vi "GetAlazar_SaveToFile_25.vi"(0 "AlazarCluster":T12, 1 "Digitizer Settings":T8={"Digitizer delay (us) "=0.0, "rf points per line"=2048, "lines per plane"=128, "Samp Rate (Hz)"=100000000.0, "Additional dig delay (us)"=0.0, "Voltage Scale"=0.4, "Pre-Looks"=0, "Offset delay (us)"=0.0, "bits A/D"=8, "Avg Num"=1, "DigTimeOut"=5.0, "Rel Dig Delay"=0.0, "Dig Ch"=0, "LeCroyCluster"={"LeCroy Channels"=[TRUE, FALSE, FALSE, FALSE], "LC read pt offset"=0.0, "Sweep Avg"=FALSE}, "Main Digitizer"=enum."NI Digitizer", "Dig Config"=enum."Single channel", "Digitizer ID Cluster"={"Acqiris/Alazar/SP ID"=[], "NI Instr Handles"=[], "LeCroy VISA"="", "GaGe Handle"={"Handle"=0, "Sample size"=0, "Resolution"=0, "Offset"=0, "Channels"=0, "Boards"=0}, "ATS Ref"="ATS9350", "Acqiris Address"=["PCI::INSTR0"], "ADQRef"=refnum, "adq_cu_ptr"=refnum}, "Trigger Settings"={"Trig Source"=1, "Trig Coupling"=0, "Trig Slope"=0, "Level (mV)"=1500.0}, "Bulk Acq"=FALSE, "Bulk Start Indexes"=[], "Data Ref RF"=refnum, "NI ID/Channel"=[], "Total Dig CH"=1, "Xtra Ann Trig delay (us)"=10.0, "Fix Z Delay?"=FALSE, "One Way Transmission?"=FALSE, "Data Ref Log"=refnum} {"Trigger Settings"."Trig Slope" items=["Positive", "Negative"]; "Trigger Settings"."Level (mV)" format="%.2f"; "Trigger Settings"."Trig Coupling" items=["DC 1 MOhm", "AC 1 MOhm", "DC 50 Ohm", "AC 50 Ohm"]; "Trigger Settings"."Trig Source" items=["Chan 1", "External"]; "Rel Dig Delay" format="%.2f"; "DigTimeOut" format="%.2f"; "Avg Num" min=1; "Offset delay (us)" format="%.2f"; "Additional dig delay (us)" format="%.2f"; "Digitizer delay (us)" format="%.2f"}, 5 "Ann Array Params":T1={"Synth Foc?"=FALSE, "Focal Zones"=41, "Switch T/R"=0, "Trans Geometry (mm)"={"Transducer"=0, "Geo Focus"=12.0, "a (radius)"=3.0, "# of rings"=5, "kerf space "=0.1, "Center Freq"=12.0}, "Sub Ap Excite?"=FALSE, "Full Array Scan?"=FALSE, "Xmt/Rcv"={"XMIT"=[TRUE, TRUE, TRUE, TRUE, TRUE], "RCV"=[TRUE, TRUE, TRUE, TRUE, TRUE]}, "PulseSpacing (us)"=0.0, "Xmit Ring"=0, "XMIT CHS"=0, "RCV CHS"=0, "GPU?"=FALSE, "Save TIFF?"=FALSE, "downfactor"=1, "RCV 1CH"=0} {"RCV 1CH" items=["All", "1", "2", "3", "4", "5"]; "Trans Geometry (mm)"."Transducer" items=["6D 12R 40 MHz"=0, "10D 31R 20 MHz"=1, "10D 23R 20 MHz"=2, "6D 23R 40 MHz"=3, "4.5D 10.7R 40 MHz"=4, "9D 23.5R 20 MHz"=5, "9D 25.8R 20MHz"=6, "Enter"=99]; "Switch T/R" min=1 max=5 step=1}, 6 "Motion Settings":T4={"No Motion?"=FALSE, "Motion System"=enum."NI 735x", "Motion Bd ID"=1, "Motion Profile"="SMAC1", "# Axis"=1, "Reverse Z axis?"=TRUE, "SMAC Axis"=0, "scan pair"=enum."y-(x) scan", "RT fps"=6.0, "Steps per mm"=[1000, 1000, 1000, 1000], "Motor Parameters"={"velocity ct/s"=[10000.0, 10000.0, 10000.0, 50000.0], "accel ct/s^2"=[50000.0, 50000.0, 50000.0, 200000.0]}, "One Way Scan"=FALSE, "Reverse One Way Scan"=FALSE, "Global Position (mm)"=[], "Plane"=0, "Distance between\nscan lines (um)"=0.0, "Distance between\nscan planes (um)"=0.0, "number of scan planes"=1, "Total steps in line"=0, "Xtra plane\ndistance  (um)"=100, "Xtra planes "=1, "Add Axis"=FALSE, "overshoot cts"=200, "BKPT Shift"=0, "Scan Start Time (ms)"=0, "ESP VISA"="GPIB::1::INSTR", "3rd Axis"=1, "GL Ref Out"=refnum, "Galil Address"=""} {"3rd Axis" items=["x", "y", "z", "w"]; "Xtra planes" min=1; "Xtra plane\ndistance  (um)" min=0; "Distance between\nscan planes (um)" format="%.2f"; "Distance between\nscan lines (um)" format="%.2f"; "SMAC Axis" items=["None"=0, "Axis 1"=1, "Axis 2"=2, "Axis 3"=3, "Axis 4"=4, "Axis 5"=5, "Axis 6"=6, "Axis 7"=7, "Axis 8"=8, "Vector Space 1"=17, "Vector Space 2"=18, "Vector Space 3"=19, "Vector Space 4"=20]; "Motion Bd ID" min=1 max=32 step=1}, 7 "errorin":errorcluster, 8 "File Array":string[](array[string]), 10 "lines per plane":i32, 15 "Reverse?":bool) -> (17 "Raw VGain (scale)":dbl, 18 "Gain Array":T13(array[cluster]), 21 "VGain (dB)":dbl, 27 "error out":errorcluster)   [LabVIEW 2022 SP3]
uses:
  Motion Controllers/-MotionRoutines/MotionGlobals.vi
  -ScanSystem/DataHandling/ReverseData.vi
  -DigitizerRoutines/DigitizerSettings.ctl
  -DigitizerRoutines/DigitizerID.ctl
  -DigitizerRoutines/Digitizer.ctl
  Motion Controllers/NI_controller/-NI_MotionRoutines/MotionSys.ctl
  Motion Controllers/-MotionRoutines/ScanAxis.ctl
  Motion Controllers/NI_controller/-NI_MotionRoutines/MotionParameters.ctl
  Annular Array/-AnnularRoutines/ArrayGeometry.ctl
  Annular Array/-AnnularRoutines/TransGeometry.ctl
  Annular Array/-AnnularRoutines/AnnularArray.ctl
  -DigitizerRoutines/DigConfig.ctl
  Motion Controllers/-MotionRoutines/3rdAxis.ctl
  C:/Windows/System32/ADQAPI_dotNet_helper.dll
panel:
  in  "Channel (0) 2":i32
  out "read time":u32
  out "save time":u32
  out "Numeric":i32
  # "1-D and 2-D B scan settings"
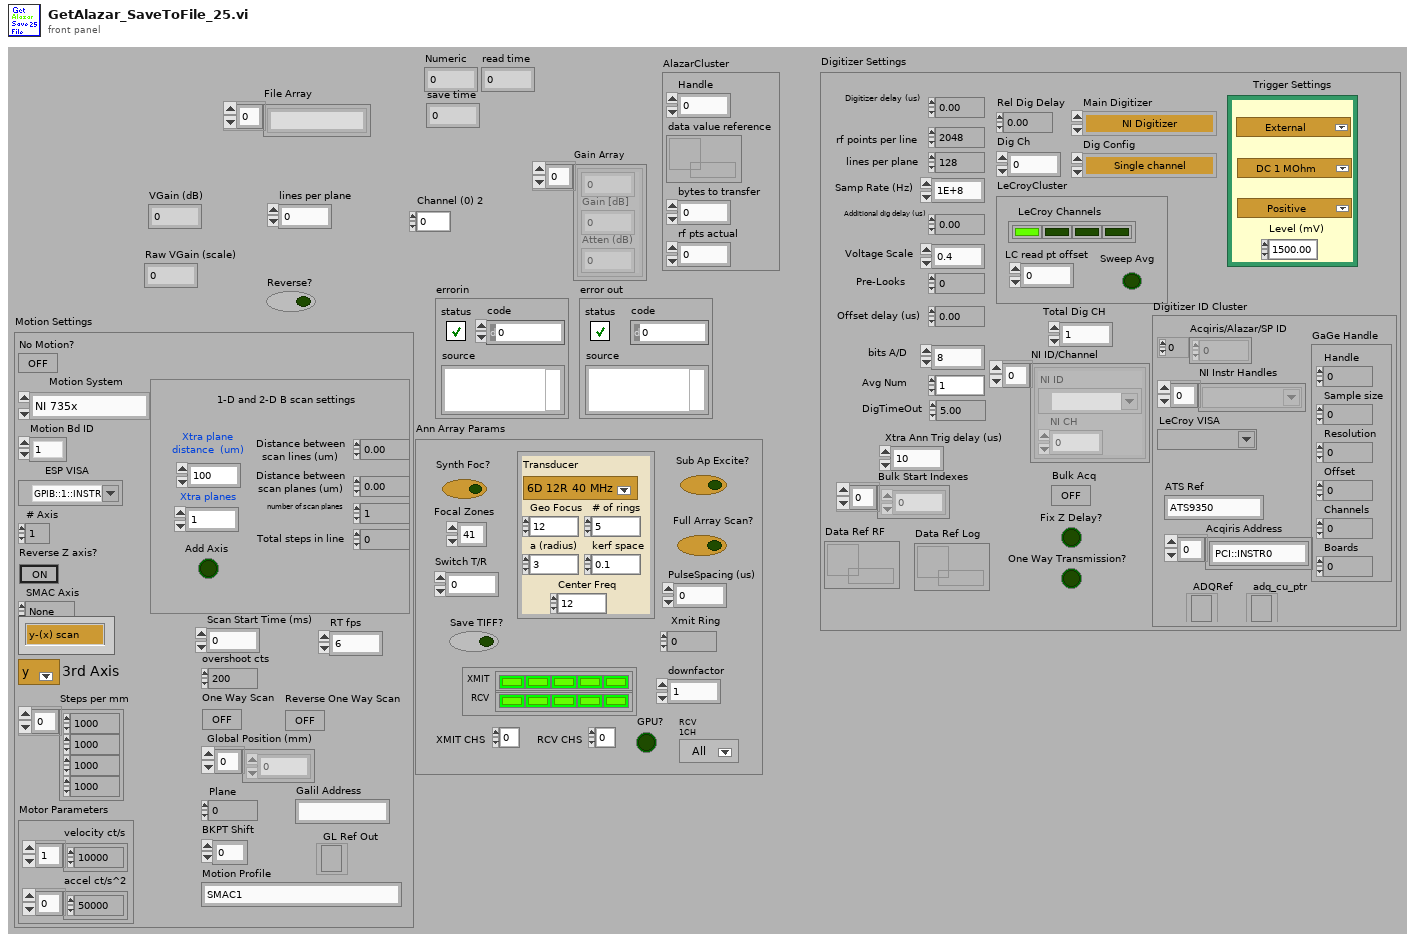
[diagram p1: front panel]
types:
  T1 = typedef "AnnularArray.ctl" = cluster{"Synth Foc?":bool, "Focal Zones":i16, "Switch T/R":i16, "Trans Geometry (mm)":T2, "Sub Ap Excite?":bool, "Full Array Scan?":bool, "Xmt/Rcv":cluster{"XMIT":bool[], "RCV":bool[]}, "PulseSpacing (us)":sgl, "Xmit Ring":i32, "XMIT CHS":u8, "RCV CHS":u8, "GPU?":bool, "Save TIFF?":bool, "downfactor":i32, "RCV 1CH":u16}
  T2 = typedef "TransGeometry.ctl" = cluster{"Transducer":T3, "Geo Focus":dbl, "a (radius)":dbl, "# of rings":i32, "kerf space ":dbl, "Center Freq":dbl}
  T3 = typedef "ArrayGeometry.ctl" = u16
  T4 = typedef "MotionParameters.ctl" = cluster{"No Motion?":bool, "Motion System":T5, "Motion Bd ID":u8, "Motion Profile":string, "# Axis":i8, "Reverse Z axis?":bool, "SMAC Axis":u16, "scan pair":T6, "RT fps":sgl, "Steps per mm":i32[], "Motor Parameters":cluster{"velocity ct/s":dbl[], "accel ct/s^2":dbl[]}, "One Way Scan":bool, "Reverse One Way Scan":bool, "Global Position (mm)":dbl[], "Plane":i32, "Distance between\nscan lines (um)":sgl, "Distance between\nscan planes (um)":sgl, "number of scan planes":i32, "Total steps in line":i32, "Xtra plane\ndistance  (um)":i32, "Xtra planes ":i32, "Add Axis":bool, "overshoot cts":i32, "BKPT Shift":i32, "Scan Start Time (ms)":u32, "ESP VISA":refnum<visa-resource-name>, "3rd Axis":T7, "GL Ref Out":refnum<k7>, "Galil Address":string}
  T5 = typedef "MotionSys.ctl" = enum16{"MM3000", "NI 735x", "Newport ESP", "No Motion Card", "Galil"}
  T6 = typedef "ScanAxis.ctl" = enum16{"y-(x) scan", "x-(y) scan", "z-(x) scan", "z-(y) scan", "y-(z) scan", "x-(z) scan", "w-(x) scan", "w-(y) scan", "w-(z) scan", "x-(w) scan", "y-(w) scan", "z-(w) scan"}
  T7 = typedef "3rdAxis.ctl" = u16
  T8 = typedef "DigitizerSettings.ctl" = cluster{"Digitizer delay (us) ":dbl, "rf points per line":i32, "lines per plane":i32, "Samp Rate (Hz)":dbl, "Additional dig delay (us)":dbl, "Voltage Scale":dbl, "Pre-Looks":i32, "Offset delay (us)":dbl, "bits A/D":i8, "Avg Num":i32, "DigTimeOut":sgl, "Rel Dig Delay":sgl, "Dig Ch":i32, "LeCroyCluster":cluster{"LeCroy Channels":bool[], "LC read pt offset":dbl, "Sweep Avg":bool}, "Main Digitizer":T9, "Dig Config":T10, "Digitizer ID Cluster":T11, "Trigger Settings":cluster{"Trig Source":u16, "Trig Coupling":u16, "Trig Slope":u16, "Level (mV)":dbl}, "Bulk Acq":bool, "Bulk Start Indexes":i32[], "Data Ref RF":refnum<data-value>, "NI ID/Channel":cluster{"NI ID":refnum<k15>, "NI CH":i32}[], "Total Dig CH":i32, "Xtra Ann Trig delay (us)":dbl, "Fix Z Delay?":bool, "One Way Transmission?":bool, "Data Ref Log":refnum<data-value>}
  T9 = typedef "Digitizer.ctl" = enum16{"Acqiris Digitizer", "NI Digitizer", "LeCroy", "GaGe", "AlazarTech", "No Digitizer", "Teledyne"}
  T10 = typedef "DigConfig.ctl" = enum16{"Single channel", "2 Chans w/ 2 Acqiris", "2 Chans w/ 1 Acqiris", "5-CH Pulser New", "5-CH pulser w/ ann array", "5-pass style ann array", "Empty"}
  T11 = typedef "DigitizerID.ctl" = cluster{"Acqiris/Alazar/SP ID":u32[], "NI Instr Handles":refnum<k15>[], "LeCroy VISA":refnum<visa-resource-name>, "GaGe Handle":cluster{"Handle":u32, "Sample size":u32, "Resolution":i32, "Offset":i32, "Channels":u32, "Boards":u32}, "ATS Ref":string, "Acqiris Address":string[], "ADQRef":refnum<k24>, "adq_cu_ptr":refnum<k24>}
  T12 = cluster{"Handle":u32, "data value reference":refnum<data-value>, "bytes to transfer":u32, "rf pts actual":u32}
  T13 = cluster{sgl, "Gain [dB]  ":sgl, "Atten (dB)":sgl}[]
  T14 = cluster{"wfm":i16[][], "max queue size (-1, unlimited)":i32}
  T15 = cluster{sgl, "Gain [dB]  ":sgl, "Atten (dB)":sgl}
  T16 = enum16{"open", "replace", "create", "open or create", "replace or create", "replace or create with confirmation"}
  T17 = enum16{"big-endian, network order", "native, host order", "little-endian"}
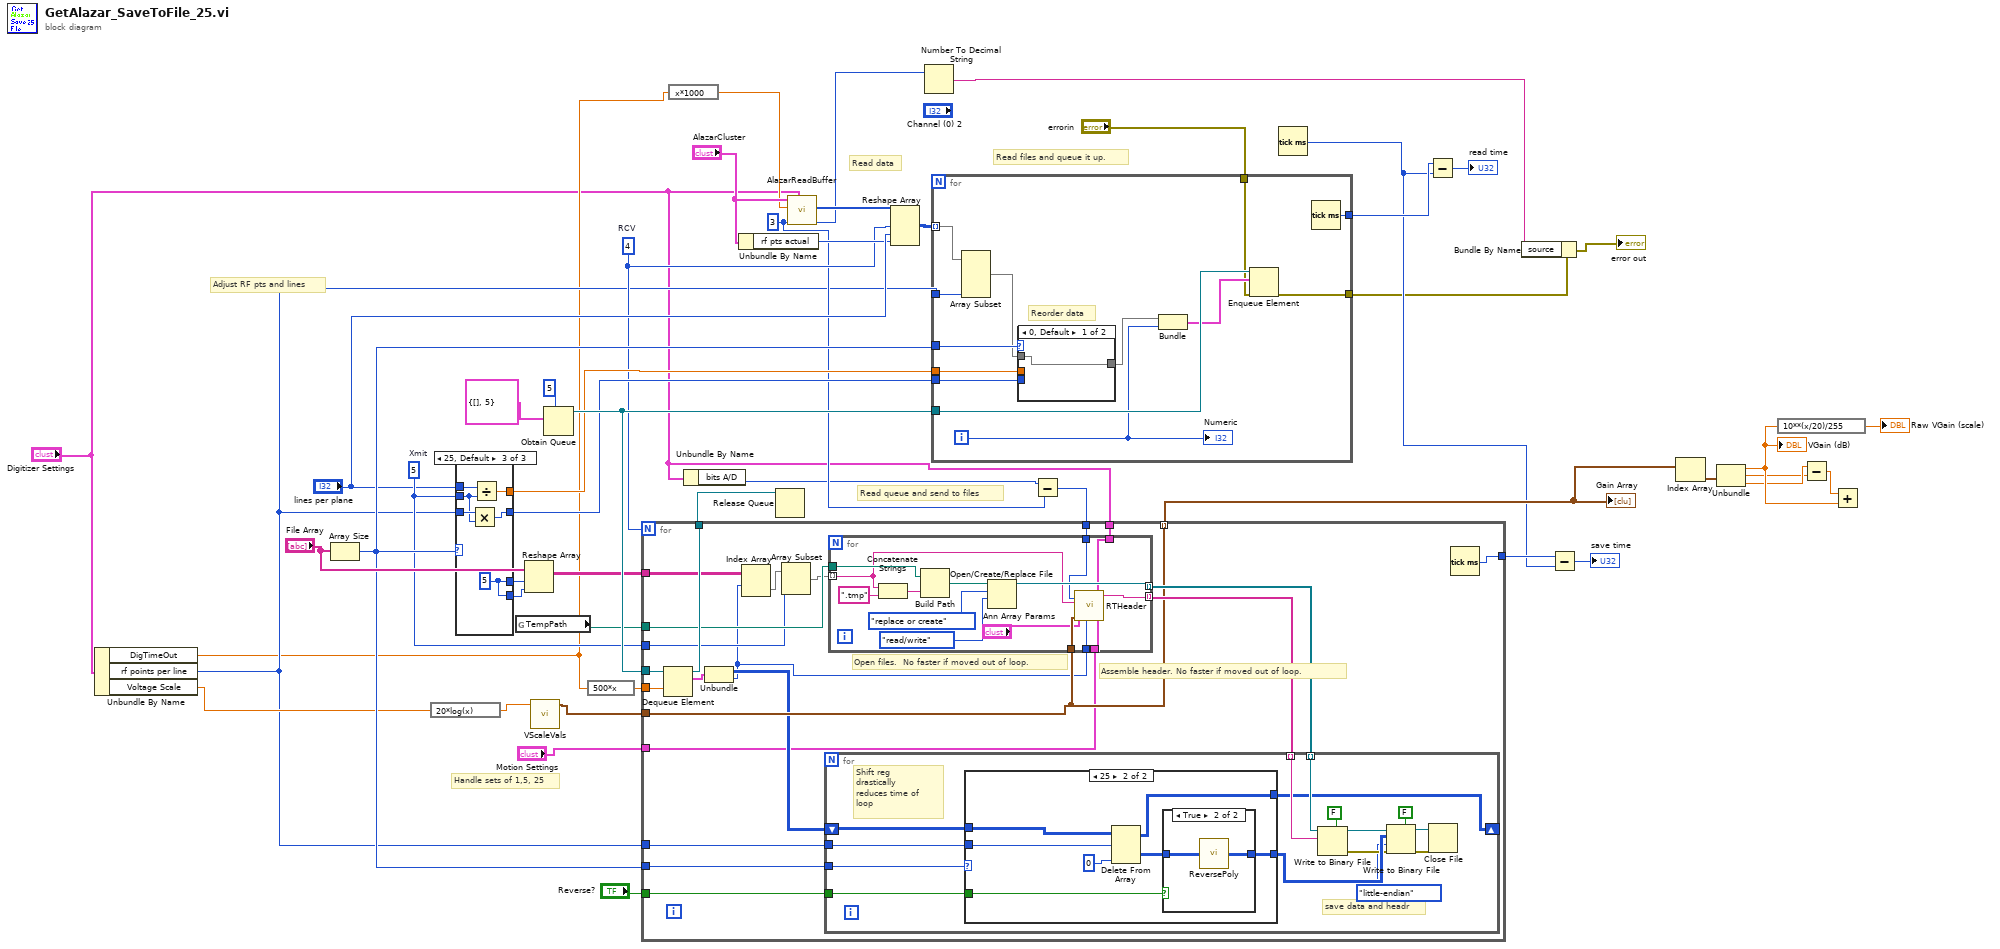
[diagram p0: block diagram]
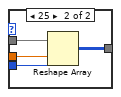
[diagram p2: hidden frame]
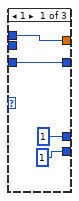
[diagram p3: hidden frame]
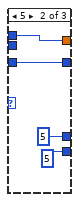
[diagram p4: hidden frame]
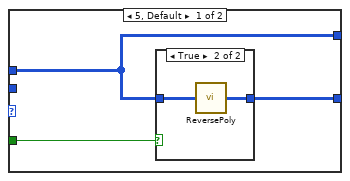
[diagram p5: hidden frame]
diagram:
  w8 = u16 3 ("Extra Shift")
  w21 = 5  # Xmit
  w15 = 4  # RCV
  # "Read data"
  # "Adjust RF pts and lines"
  # "Handle sets of 1,5, 25"
  # "Read files and queue it up."
  # "Read queue and send to files"
  n1 = Unbundle By Name("Digitizer Settings") -> ("DigTimeOut"=w3:sgl, "rf points per line"=w5:i32, "Voltage Scale"=w6:dbl)
  n2 = Array Size(array="File Array") -> (size(s)=w26:i32)
  n3 = expression code="20*log(x)"(w6) -> (w23:dbl)
  n4 = case shown="25, Default" w26 {
    tunnel: [1 5 w63] -> w31
    tunnel: [w52 w56 w59] -> w28
    tunnel: w5 -> [w52 w56 w60]
    tunnel: [w51 w55 w61] -> w29
    tunnel: "lines per plane" -> [w51 w55 w62]
    tunnel: [1 5 w63] -> w30
    tunnel: w21 -> [_ _ w58]
    frame 1 {
    }
    frame 5 {
    }
    frame 25, Default {
      w63 = 5
      n5 = Multiply(x=w60, y=w58) -> (x*y=w59:i32)
      n6 = Divide(x=w62, y=w58) -> (x/y=w61:dbl)
    }
  }
  n7 = global read "MotionGlobals.vi" "TempPath"() -> (w24:path)
  n8 = Reshape Array("File Array", w31, w30) -> (w25:string[][])
  n9 = call "VScaleVals.vi"("Full Scale"=w23) -> ("Voltage Scale"=w22:T15)  [unwired: 8 in, 2 out]
  n10 = Obtain Queue(max queue size (-1, unlimited)=5, element data type=T14 {"wfm"=[], "max queue size (-1, unlimited)"=5}) -> (queue out=w41:refnum<queue>)  [unwired: 3 in, 2 out]
  n11 = expression code="500*x"(w3) -> (w27:sgl)
  n12 = expression code="x*1000"(w3) -> (w13:sgl)
  n13 = Unbundle By Name("Digitizer Settings") -> ("bits A/D"=w4:i8)
  n14 = Unbundle By Name("AlazarCluster") -> ("rf pts actual"=w17:u32)
  n15 = call "AlazarReadBuffer.vi"("Digitizer Settings"="Digitizer Settings", "Extra Shift"=w8, "time out"=w13, "AlazarCluster"="AlazarCluster") -> ("Return Code"=w9:u32, "Data Array"=w18:i16[])  [unwired: 5 in, 1 out]
  n16 = Reshape Array(w18, w15, "lines per plane", w17) -> (w16:i16[][][])
  n17 = Number To Decimal String(number=w9) -> (decimal integer string=w11:string)  [unwired: 1 in]
  n18 = for {
    tunnel: w41 -> [w76]
    tunnel: [w74] -> w39
    tunnel: [w73] -> w12
    tunnel: w26 -> [w72]
    tunnel: w29 -> [w71]
    tunnel: w28 -> [w70]
    tunnel: w16 -> [w68] mode=indexing
    tunnel: w5 -> [w67]
    tunnel: "errorin" -> [w64]
    i -> [w65]
    # "Reorder data"
    n19 = Array Subset(array=w68, length (col)=w67) -> (w66:i16[][])  [unwired: 3 in]
    n20 = case shown="0, Default" w72 {
      tunnel: w70 -> [_ w81]
      tunnel: w66 -> [w77 w80]
      tunnel: [w77 w79] -> w69
      tunnel: w71 -> [_ w78]
      frame 0, Default {
      }
      frame 25 {
        n21 = Reshape Array(w80, w78, w81) -> (w79:i16[][])
      }
    }
    n22 = Bundle(w69, w65) -> (w75:cluster{i16[][], i32})  [unwired: 1 in]
    n23 = Enqueue Element(queue=w76, element=w75, error in (no error)=w64) -> (error out=w73:errorcluster)  [unwired: 1 in, 2 out]
    n24 = Tick Count (ms)() -> (millisecond timer value=w74:u32)
    "Numeric" <- w65
  }
  n25 = Subtract(x=w4, y=w8) -> (x-y=w7:u16)
  n26 = for {
    N: w15 -> [_]
    tunnel: w5 -> [w102]
    tunnel: "Reverse?" -> [w97]
    tunnel: [w86] -> w42 mode=indexing
    tunnel: w41 -> [w101]
    tunnel: [w99] -> w33
    tunnel: [w98] -> w38
    tunnel: w26 -> [w96]
    tunnel: w27 -> [w95]
    tunnel: w25 -> [w90]
    tunnel: w24 -> [w93]
    tunnel: w7 -> [w92]
    tunnel: w21 -> [w87]
    tunnel: w22 -> [w86]
    tunnel: "Digitizer Settings" -> [w84]
    tunnel: "Motion Settings" -> [w83]
    # "Open files.  No faster if moved out of loop."
    # "Assemble header. No faster if moved out of loop."
    n27 = Dequeue Element(queue=w101, timeout in ms (-1)=w95) -> (queue out=w99:refnum<queue>, element=w100:T14)  [unwired: 1 in, 2 out]
    n28 = Unbundle(w100) -> ("wfm"=w85:i16[][], "max queue size (-1, unlimited)"=w82:i32)
    n29 = Index Array(array=w90, index (row)=w82) -> (element=w88:string[])  [unwired: 1 in]
    n30 = Array Subset(array=w88, length=w87) -> (w89:string[])  [unwired: 1 in]
    n31 = for {
      tunnel: w89 -> [w110] mode=indexing
      tunnel: [w112] -> w94 mode=indexing
      tunnel: w93 -> [w111]
      tunnel: w86 -> [w109]
      tunnel: w92 -> [w108]
      tunnel: [w107] -> w91 mode=indexing
      tunnel: w84 -> [w106]
      tunnel: w83 -> [w105]
      tunnel: w82 -> [w104]
      n32 = Concatenate Strings(w110, ".tmp") -> (w113:string)
      n33 = Build Path(base path=w111, name or relative path=w113) -> (appended path=w117:path)
      n34 = Open/Create/Replace File(file path (use dialog)=w117, operation (0:open)=T16."replace or create", access (0:read/write)=enum16{"read/write", "read-only", "write-only"}."read/write") -> (refnum out=w112:refnum<file>)  [unwired: 1 in, 4 out]
      n35 = call "RTHeader.vi"("Motion Settings"=w105, "Dig Word Size"=w108, "Pulser Channel"=w104, "Digitizer Settings"=w106, "Votage scaling"=w109, "Ann Array Params"="Ann Array Params", "File Name In"=w110) -> ("Header String Out"=w107:string)  [unwired: 3 in, 1 out]
    }
    n36 = for {
      tunnel: w91 -> [w130] mode=indexing
      tunnel: w97 -> [w129]
      tunnel: w94 -> [w122] mode=indexing
      tunnel: w102 -> [w128]
      tunnel: w96 -> [w126]
      shift-right: [w119] -> _
      shift-left: w85 -> [w127]
      # "Shift reg drastically reduces time of loop"
      # "save data and headr"
      n37 = case shown="25" w126 {
        tunnel: w129 -> [w135 w143]
        tunnel: [w134 w144] -> w125
        tunnel: w128 -> [_ w140]
        tunnel: w127 -> [w133 w142]
        tunnel: [w133 w141] -> w119
        frame 5, Default {
          n38 = case shown="True" w135 {
            tunnel: [w136 w138] -> w134
            tunnel: w133 -> [w136 w137]
            frame False {
            }
            frame True {
              n39 = call-poly "ReversePoly.vi"("Array in"=w137) -> ("Array out"=w138:i16[][])
            }
          }
        }
        frame 25 {
          n40 = Delete From Array(array=w142, length=w140, index (col)=0 ("index (row)")) -> (deleted portion=w145:i16[][], array with subset deleted=w141:i16[][])  [unwired: 1 in]
          n41 = case shown="True" w143 {
            tunnel: [w146 w148] -> w144
            tunnel: w145 -> [w146 w147]
            frame False {
            }
            frame True {
              n42 = call-poly "ReversePoly.vi"("Array in"=w147) -> ("Array out"=w148:i16[][])
            }
          }
        }
      }
      n43 = Write to Binary File(file (use dialog)=w122, data=w130, 5:FALSE ("prepend array or string size? (T)")) -> (refnum out=w121:refnum<file>, error out=w120:errorcluster)  [unwired: 3 in, 1 out]
      n44 = Write to Binary File(file (use dialog)=w121, data=w125, error in=w120, 5:FALSE ("prepend array or string size? (T)"), 9:T17."little-endian" ("byte order (0:big-endian, network order)")) -> (refnum out=w124:refnum<file>, error out=w123:errorcluster)  [unwired: 1 in, 1 out]
      n45 = Close File(refnum=w124, error in=w123) -> ()  [unwired: 2 out]
    }
    n46 = Tick Count (ms)() -> (millisecond timer value=w98:u32)
  }
  "Gain Array" <- w42
  n47 = Release Queue(queue=w33) -> ()  [unwired: 2 in, 3 out]
  n48 = Tick Count (ms)() -> (millisecond timer value=w37:u32)
  n49 = Subtract(x=w39, y=w37) -> (x-y=→"read time":u32)
  n50 = Bundle By Name(cluster=w12, "source"=w11) -> (→"error out":errorcluster)
  n51 = Subtract(x=w38, y=w37) -> (x-y=→"save time":u32)
  n52 = Index Array(array=w42) -> (element=w49:T15)  [unwired: 1 in]
  n53 = Unbundle(w49) -> (w48:sgl, "Gain [dB]"=w46:sgl, "Atten (dB)"=w47:sgl)
  "VGain (dB)" <- w48
  n54 = expression code="10**(x/20)/255"(w48) -> (→"Raw VGain (scale)":sgl)
  n55 = Subtract(x=w47, y=w46) -> (x-y=w45:sgl)
  n56 = Add(x=w45, y=w48) -> ()  [unwired: 1 out]
